vi "Polynomial Fit Intervals.vi"   [LabVIEW 2010, in "NI_AALPro.lvlib"]
doc: "Calculates statistical intervals of the best polynomial fit for a data set (<B>X</B>, <B>Y</B>)."
uses:
  NI_AALPro.lvlib
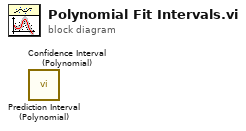
[diagram p0: block diagram]
diagram:
  n1 = call "Prediction Interval (Polynomial).vi"() -> ()  [unwired: 13 in, 3 out]
  n2 = call "Confidence Interval (Polynomial).vi"() -> ()  [unwired: 12 in, 4 out]
